vi "Shooting Power.vi"(1 "Quarter 2":bool, 2 "Half 2":bool, 3 "Full 2":bool) -> (0 "Value":T1=enum."Forward")   [LabVIEW 2013]
uses:
  <vilib>/Rock Robotics/WPI/Solenoid/WPI_SolenoidValue.ctl
panel:
  out "Half":bool
  out "Full":bool
  out "Quarter":bool
  in  "Time to a full shoot":dbl
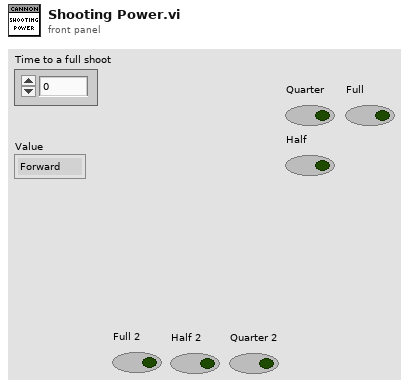
[diagram p1: front panel]
types:
  T1 = typedef "WPI_SolenoidValue.ctl" = enum16{"Off", "On", "Forward", "Reverse"}
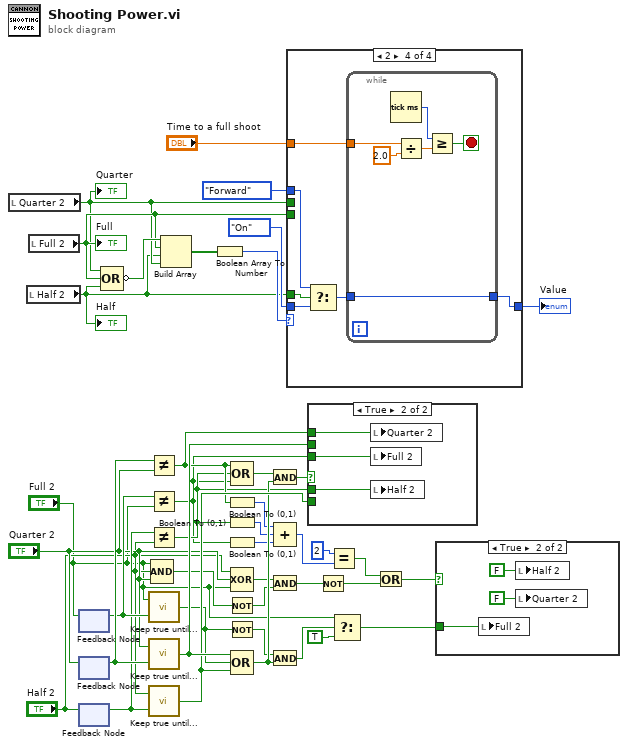
[diagram p0: block diagram]
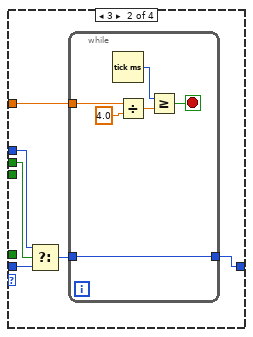
[diagram p3: hidden frame]
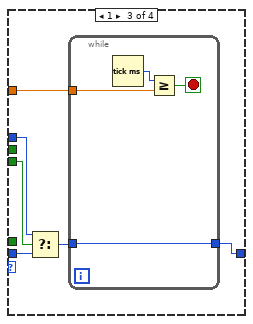
[diagram p4: hidden frame]
diagram:
  n1 = local read "Quarter 2"() -> (w2:bool)
  "Quarter" <- w2
  n2 = local read "Half 2"() -> (w1:bool)
  "Half" <- w1
  n3 = local read "Full 2"() -> (w3:bool)
  "Full" <- w3
  n4 = feedback #1() -> (w36:bool)  [unwired: 1 in]
  n5 = feedback-in #1("Full 2") -> ()
  n6 = feedback #2() -> (w37:bool)  [unwired: 1 in]
  n7 = feedback-in #2("Quarter 2") -> ()
  n8 = feedback #3() -> (w35:bool)  [unwired: 1 in]
  n9 = feedback-in #3("Half 2") -> ()
  n10 = Compound Arithmetic op=OR(w2, w3, w1) -> (invert w5:bool)
  n11 = Not Equal?(x=w37, y="Quarter 2") -> (x != y?=w23:bool)
  n12 = Not Equal?(x=w36, y="Full 2") -> (x != y?=w21:bool)
  n13 = Not Equal?(x=w35, y="Half 2") -> (x != y?=w22:bool)
  n14 = call "Keep true until....vi"("Changer"=w36, "Keep"="Full 2") -> ("Value"=w32:bool)
  n15 = call "Keep true until....vi"("Changer"=w37, "Keep"="Quarter 2") -> ("Value"=w39:bool)
  n16 = call "Keep true until....vi"("Changer"=w35, "Keep"="Half 2") -> ("Value"=w38:bool)
  n17 = Compound Arithmetic op=AND("Full 2", "Half 2", "Quarter 2") -> (w30:bool)
  n18 = Build Array(w5, w3, w1, w2) -> (w4:bool[])
  n19 = Boolean Array To Number(Boolean array=w4) -> (number=w6:u32)
  n20 = Boolean To (0,1)(Boolean=w23) -> (0, 1=w20:i16)
  n21 = Boolean To (0,1)(Boolean=w22) -> (0, 1=w19:i16)
  n22 = Boolean To (0,1)(Boolean=w21) -> (0, 1=w18:i16)
  n23 = Not(x=w30) -> (.not. x?=w29:bool)
  n24 = Not(x=w32) -> (.not. x?=w33:bool)
  n25 = Compound Arithmetic op=OR(w23, w22, w21) -> (w41:bool)
  n26 = Compound Arithmetic op=XOR("Half 2", "Quarter 2", "Full 2") -> (w28:bool)
  n27 = Compound Arithmetic op=OR(w39, w32, w38) -> (w34:bool)
  n28 = And(x=w41, y=w34) -> (x .and. y?=w25:bool)
  n29 = And(x=w28, y=w29) -> (x .and. y?=w14:bool)
  n30 = And(x=w33, y=w34) -> (x .and. y?=w31:bool)
  n31 = Compound Arithmetic op=ADD(w20, w19, w18) -> (w17:i16)
  n32 = case shown="2" w6 {
    tunnel: [w42 w45 w58 w66] -> w10
    tunnel: "Time to a full shoot" -> [_ w48 w56 w70]
    tunnel: WPI_SolenoidValue."Forward" ("Value") -> [_ w47 w60 w69]
    tunnel: WPI_SolenoidValue."On" ("Value") -> [w42 w46 w59 w68]
    tunnel: w1 -> [_ _ _ w65]
    tunnel: w2 -> [_ w43 _ _]
    tunnel: w3 -> [_ _ w55 _]
    frame 0, Default {
    }
    frame 3 {
      n33 = Select(t=w47, s=w43, f=w46) -> (s? t:f=w44:T1)
      n34 = while {
        tunnel: w48 -> [w52]
        tunnel: [w49] -> w45
        tunnel: w44 -> [w49]
        stop <- w53 stop-if-true
        n35 = Tick Count (ms)() -> (millisecond timer value=w54:u32)
        n36 = Divide(x=w52, y=4.0) -> (x/y=w50:dbl)
        n37 = Greater Or Equal?(x=w54, y=w50) -> (x >= y?=w53:bool)
      }
    }
    frame 1 {
      n38 = Select(t=w60, s=w55, f=w59) -> (s? t:f=w57:T1)
      n39 = while {
        tunnel: [w62] -> w58
        tunnel: w57 -> [w62]
        tunnel: w56 -> [w61]
        stop <- w63 stop-if-true
        n40 = Tick Count (ms)() -> (millisecond timer value=w64:u32)
        n41 = Greater Or Equal?(x=w64, y=w61) -> (x >= y?=w63:bool)
      }
    }
    frame 2 {
      n42 = Select(t=w69, s=w65, f=w68) -> (s? t:f=w67:T1)
      n43 = while {
        tunnel: w70 -> [w73]
        tunnel: w67 -> [w71]
        tunnel: [w71] -> w66
        stop <- w75 stop-if-true
        n44 = Tick Count (ms)() -> (millisecond timer value=w76:u32)
        n45 = Divide(x=w73, y=2.0) -> (x/y=w72:dbl)
        n46 = Greater Or Equal?(x=w76, y=w72) -> (x >= y?=w75:bool)
      }
    }
  }
  "Value" <- w10
  n47 = case shown="True" w25 {
    tunnel: w39 -> [_ _]
    tunnel: w38 -> [_ _]
    tunnel: w22 -> [_ w79]
    tunnel: w23 -> [_ w78]
    tunnel: w21 -> [_ w77]
    frame False {
    }
    frame True {
      n48 = local write "Quarter 2"(w78) -> ()
      n49 = local write "Full 2"(w77) -> ()
      n50 = local write "Half 2"(w79) -> ()
    }
  }
  n51 = Not(x=w14) -> (.not. x?=w13:bool)
  n52 = Equal?(x=i16 2, y=w17) -> (x = y?=w12:bool)
  n53 = Select(t="Full 2", s=w31, f=TRUE) -> (s? t:f=w24:bool)
  n54 = Or(x=w12, y=w13) -> (x .or. y?=w15:bool)
  n55 = case shown="True" w15 {
    tunnel: w24 -> [_ w80]
    frame False {
    }
    frame True {
      n56 = local write "Full 2"(w80) -> ()
      n57 = local write "Half 2"(FALSE ("Right")) -> ()
      n58 = local write "Quarter 2"(FALSE ("Left")) -> ()
    }
  }
